vi "Save Unique File Certain Time.vi"(6 "Save?":bool, 7 "Waveform":waveform(dbl), 8 "error in (no error)":errorcluster, 9 "Seconds In File":dbl, 11 "File Parameters":T1) -> (0 "error out":errorcluster, 2 "current file path out":path, 3 "last finished file path out":path)   [LabVIEW 2024]
uses:
  <vilib>/Waveform/WDTOps.llb/WDT Waveform Duration DBL.vi
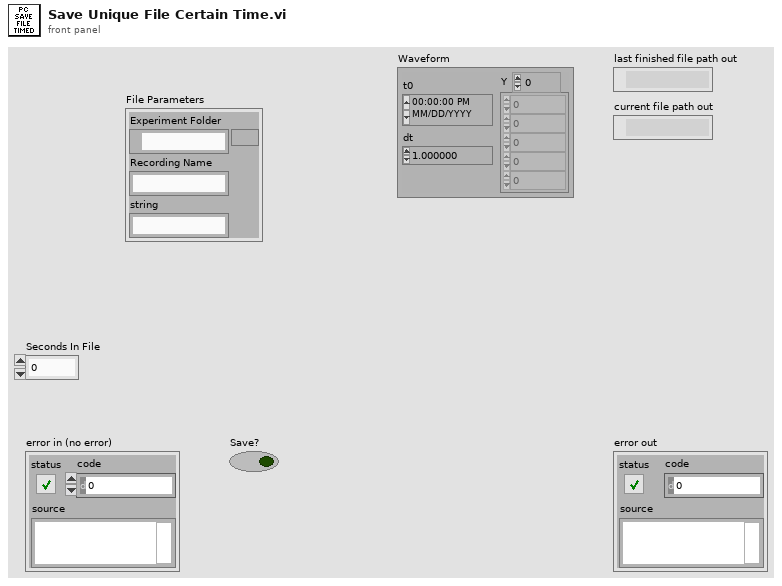
[diagram p1: front panel]
types:
  T1 = cluster{"Experiment Folder":path, "Recording Name":string, "string":string}
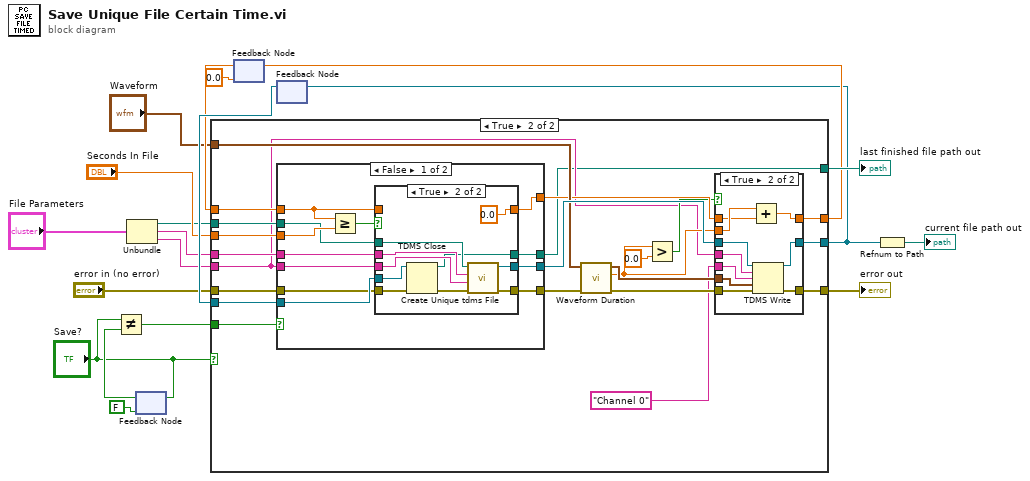
[diagram p0: block diagram]
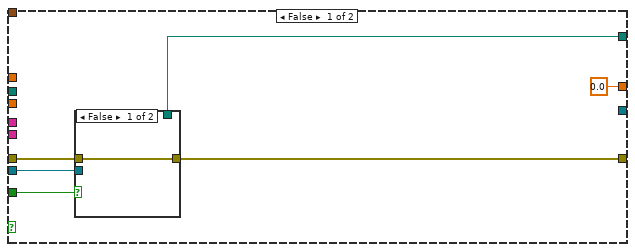
[diagram p2: hidden frame]
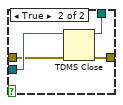
[diagram p3: hidden frame]
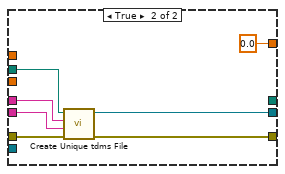
[diagram p6: hidden frame]
diagram:
  n1 = Unbundle("File Parameters") -> ("Experiment Folder"=w6:path, "Recording Name"=w5:string, "string"=w4:string)
  n2 = feedback #1(FALSE ("Save?")) -> (w9:bool)
  n3 = Not Equal?(x="Save?", y=w9) -> (x != y?=w7:bool)
  n4 = feedback-in #1("Save?") -> ()
  n5 = feedback #2(0.0 ("duration")) -> (w15:dbl)
  n6 = feedback #3() -> (w17:refnum<k34>)  [unwired: 1 in]
  n7 = case shown="True" "Save?" {
    tunnel: w7 -> [w24 w52]
    tunnel: w6 -> [_ w51]
    tunnel: w5 -> [_ w50]
    tunnel: w4 -> [_ w34]
    tunnel: "Waveform" -> [_ w46]
    tunnel: "error in (no error)" -> [w22 w48]
    tunnel: [_ w47] -> w2
    tunnel: [0.0 w42] -> w13
    tunnel: w15 -> [_ w41]
    tunnel: "Seconds In File" -> [_ w40]
    tunnel: w17 -> [w23 w39]
    tunnel: [w21 w33] -> w18
    tunnel: [w20 w32] -> w19
    frame False {
      n8 = case shown="False" w24 {
        tunnel: w23 -> [_ w30]
        tunnel: w22 -> [w26 w29]
        tunnel: [w26 w28] -> w21
        tunnel: [_ w27] -> w20
        frame False {
        }
        frame True {
          n9 = TDMS Close(8:w29, 11:w30) -> (0:w28:errorcluster, 3:w27:path)
        }
      }
    }
    frame True {
      n10 = case shown="False" w52 {
        tunnel: w51 -> [w72 w97]
        tunnel: w50 -> [w73 w96]
        tunnel: w34 -> [w74 w95]
        tunnel: [w71 w94] -> w49
        tunnel: [w70 w93] -> w45
        tunnel: w48 -> [w69 w92]
        tunnel: w41 -> [w68 _]
        tunnel: w40 -> [w77 _]
        tunnel: w39 -> [w75 _]
        tunnel: [w67 0.0 ("duration")] -> w38
        tunnel: [w66 _] -> w32
        frame False {
          n11 = Greater Or Equal?(x=w68, y=w77) -> (x >= y?=w76:bool)
          n12 = case shown="True" w76 {
            tunnel: w75 -> [w80 w90]
            tunnel: w74 -> [_ w89]
            tunnel: w73 -> [_ w88]
            tunnel: w72 -> [_ w87]
            tunnel: [w80 w86] -> w71
            tunnel: [w79 w84] -> w70
            tunnel: w69 -> [w79 w83]
            tunnel: w68 -> [w78 _]
            tunnel: [w78 0.0 ("duration")] -> w67
            tunnel: [_ w81] -> w66
            frame False {
            }
            frame True {
              n13 = TDMS Close(8:w83, 11:w90) -> (0:w85:errorcluster, 3:w81:path)
              n14 = call "Create Unique tdms File.vi"("error in (no error)"=w85, "string"=w89, "Recording Name"=w88, "Experiment Folder"=w87) -> ("error out"=w84:errorcluster, "Refnum out"=w86:refnum<k34>)  [unwired: 6 in]
            }
          }
        }
        frame True {
          n15 = call "Create Unique tdms File.vi"("error in (no error)"=w92, "string"=w95, "Recording Name"=w96, "Experiment Folder"=w97) -> ("error out"=w93:errorcluster, "Refnum out"=w94:refnum<k34>)  [unwired: 6 in]
        }
      }
      n16 = call-poly <vilib>:"Waveform Duration.vi"("error in (no error)"=w45, "waveform in"=w46) -> ("error out"=w44:errorcluster, "duration"=w37:dbl, "waveform out"=w43:waveform(dbl))  [unwired: 7 in]
      n17 = Greater?(x=w37, y=0.0) -> (0:w35:bool)
      n18 = case shown="True" w35 {
        tunnel: w49 -> [w55 w65]
        tunnel: [w55 w64] -> w47
        tunnel: w44 -> [w53 w63]
        tunnel: w43 -> [_ w62]
        tunnel: w37 -> [_ w61]
        tunnel: [w54 w60] -> w42
        tunnel: w38 -> [w54 w59]
        tunnel: "Channel 0" ("channel name(s) in (Untitled)") -> [_ w58]
        tunnel: w34 -> [_ w57]
        tunnel: [w53 w56] -> w33
        frame False {
        }
        frame True {
          n19 = Add(x=w61, y=w59) -> (x+y=w60:dbl)
          n20 = TDMS Write(0:w65, 5:w57, 7:w58, 9:w62, 11:w63) -> (4:w64:refnum<k34>, 15:w56:errorcluster)  [unwired: 1 in, 2 out]
        }
      }
    }
  }
  "last finished file path out" <- w19
  "error out" <- w18
  n21 = feedback-in #2(w13) -> ()
  n22 = feedback-in #3(w2) -> ()
  n23 = Refnum to Path(1:w2) -> (0:→"current file path out":path)
